vi "ExNframeROI.vi"() -> ()   [LabVIEW 2010]
panel:
  in  "Trigger Edge":u32(ring)=1 items=["", "Positive (leading) edge", "Negative (falling) Edge"]
  in  "Trigger/Timing Mode":u32(ring)=1 items=["N/A", "FreeRun/Timed", "Single Trigger (PM only)", "Ext Sync/Strobed", "Bulb (PM only)", "Variable (PM only)", "Flash Mode (PM only)"]
  in  "Y End":u32=1 min=1 step=1
  in  "Y Start":u32=1 min=1 step=1
  in  "X Bin":u32=1 min=1 step=1
  in  "X End":u32=1 min=1 step=1
  in  "Y Bin":u32=1 min=1 step=1
  in  "X Start":u32=1 min=1 step=1
  in  "Number of Images":u32=1 min=1 step=1
  in  "Intensifier":bool
  in  "Temperature":dbl=-10.0 format="%.2f"
  in  "Exposure":dbl min=0.0 step=0.001 format="%.3f"
  out "error out":errorcluster
  in  "error in (no error)":errorcluster
  # "ExNframeROI:\nThis example sets up the camera with a given ROI, and \ncollects into a file \"number of Images\"  set by user. The \nImages are also displayed.\nNote: not all cameras support nframe."
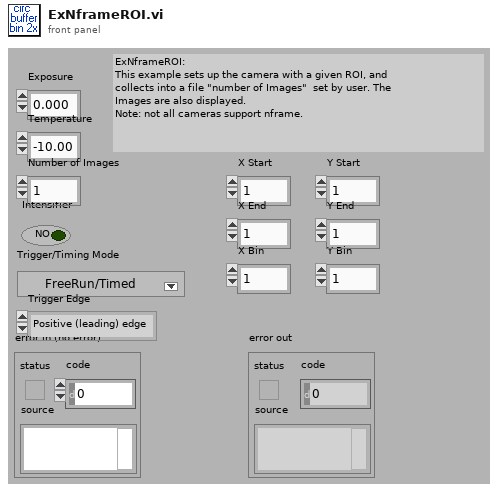
[diagram p1: front panel]
types:
  T1 = cluster{"X Start":u32, "X End":u32, "X Bin":u32, "Y Start":u32, "Y End":u32, "Y Bin":u32}
  T2 = cluster{"acquire focus mode":u32, "Exposure":dbl, "Number of Images":u32, "Software accumulation":u32}
  T3 = cluster{"Camera Handle":u32, "Pulser Handle":u32, "File Handle":u32, "Display Handle":u32, "Image Handle":u32}
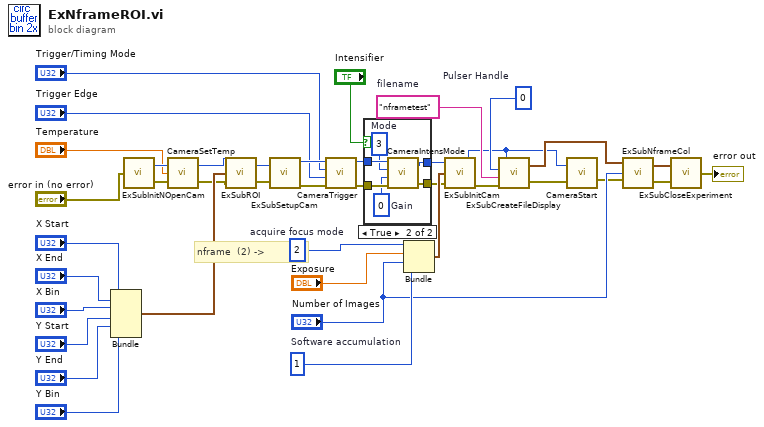
[diagram p0: block diagram]
diagram:
  w29 = u32 0  # Pulser Handle
  w31 = u32 2  # acquire focus mode
  w30 = u32 1  # Software accumulation
  w39 = "nframetest"  # filename
  # "nframe  (2) ->"
  n1 = Bundle("X Start"="X Start", "X End"="X End", "X Bin"="X Bin", "Y Start"="Y Start", "Y End"="Y End", "Y Bin"="Y Bin") -> (w14:T1)  [unwired: 1 in]
  n2 = call "ExSubInitNOpenCam.vi"("error in (no error)"="error in (no error)") -> ("Camera Handle"=w9:u32, "error out"=w8:errorcluster)
  n3 = call <userlib>:"CameraSetTemp.vi"("error in (no error)"=w8, "Temperature"="Temperature", "Camera Handle"=w9) -> ("error out"=w6:errorcluster, "Camera Handle"=w7:u32)
  n4 = call "ExSubROI.vi"("error in (no error)"=w6, "ROI"=w14, "Camera Handle"=w7) -> ("error out"=w3:errorcluster, "Camera Handle"=w4:u32)
  n5 = call "ExSubSetupCam.vi"("error in (no error)"=w3, "Camera Handle"=w4) -> ("error out"=w32:errorcluster, "Camera Handle"=w33:u32)
  n6 = call <userlib>:"CameraTrigger.vi"("error in"=w32, "Trigger Edge"="Trigger Edge", "Timing Mode"="Trigger/Timing Mode", "Camera Handle"=w33) -> ("error out"=w26:errorcluster, "Camera Handle"=w28:u32)
  n7 = case shown="True" "Intensifier" {
    tunnel: w28 -> [w41 w47]
    tunnel: [w41 w46] -> w27
    tunnel: w26 -> [w40 w45]
    tunnel: [w40 w44] -> w25
    frame False {
    }
    frame True {
      w42 = u32 0  # Gain
      w43 = u32 3  # Mode
      n8 = call <userlib>:"CameraIntensMode.vi"("error in"=w45, "Intensifier Gain"=w42, "Mode"=w43, "Camera Handle"=w47) -> ("error out"=w44:errorcluster, "Camera Handle"=w46:u32)
    }
  }
  n9 = Bundle("acquire focus mode"=w31, "Exposure"="Exposure", "Number of Images"="Number of Images", "Software accumulation"=w30) -> (w36:T2)  [unwired: 1 in]
  n10 = call "ExSubInitCam.vi"("error in (no error)"=w25, "Camera Information"=w36, "Camera Handle"=w27) -> ("error out"=w35:errorcluster, "Camera Handle"=w10:u32)
  n11 = call "ExSubCreateFileDisplay.vi"("error in (no error)"=w35, "File and Display Name"=w39, "Pulser Handle"=w29, "Camera Handle"=w10) -> ("error out"=w13:errorcluster, "Handles Out"=w11:T3)
  n12 = call <userlib>:"CameraStart.vi"("error in"=w13, "Camera Handle"=w10) -> ("error out"=w12:errorcluster)  [unwired: 1 out]
  n13 = call "ExSubNframeCol.vi"("error in (no error)"=w12, "Number of Images"="Number of Images", "Handle Cluster"=w11) -> ("error out"=w22:errorcluster, "Handle Cluster"=w23:T3)
  n14 = call "ExSubCloseExperiment.vi"("error in (no error)"=w22, "Handles In"=w23) -> ("error out"=→"error out":errorcluster)
